vi "Get_Circ_Area_Array.vi"(4 "Radius":dbl[](array[numeric])) -> (1 "Area":dbl[](array[numeric]))   [LabVIEW 2011]
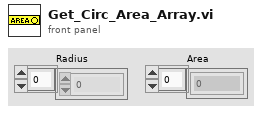
[diagram p1: front panel]
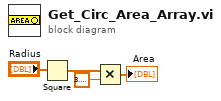
[diagram p0: block diagram]
diagram:
  n1 = Square(x="Radius") -> (x^2=w4:dbl[])
  n2 = Multiply(x=w4, y=3.141592653589793) -> (x*y=→"Area":dbl[])
